vi "Send CMD.vi"(8 "error in":errorcluster, 10 "CMD In":string, 11 "Vaisala in":refnum<class "Vaisala.lvclass">) -> (0 "error out":errorcluster, 3 "Vaisala out":refnum<class "Vaisala.lvclass">)   [LabVIEW 2014, in "Vaisala.lvclass"]
uses:
  Vaisala.lvclass
  reusable/Session APIs/Serial/Serial Session.lvclass
  Vaisala.lvclass/Vaisala.ctl
  reusable/Session APIs/Serial/Public/Get Data/Get String.vi
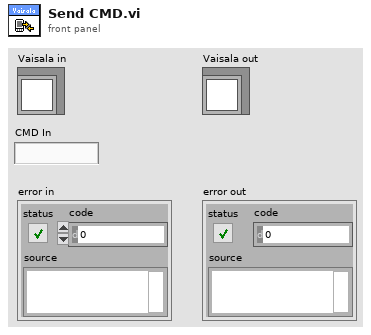
[diagram p1: front panel]
types:
  T1 = typedef "Session - Root.lvclass/Session Handle.ctl" = refnum<data-value>
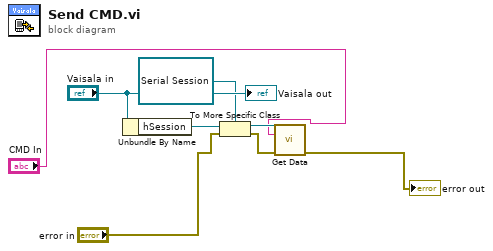
[diagram p0: block diagram]
diagram:
  n1 = Unbundle By Name("Vaisala in") -> ("hSession"=w6:T1)
  n2 = To More Specific Class(target class=refnum<data-value> refnum, reference=w6, error in="error in") -> (specific class reference=w2:refnum<data-value>, error out=w4:errorcluster)
  n3 = call-poly "Get Data.vi"("Session Handle in"=w2, "CMD"="CMD In", "error in"=w4) -> ("error out"=→"error out":errorcluster)  [unwired: 10 in, 2 out]
  "Vaisala out" <- "Vaisala in"
